vi "Knock Sensor Page Wrapper.vi"(8 "error in (no error)":errorcluster, 11 "Node Ptr":T1 format="%.0x") -> (0 "error out":errorcluster)   [LabVIEW 2015, in "Engine Simulation Toolkit System Explorer.lvlib"]
uses:
  Engine Simulation Toolkit System Explorer.lvlib
  <vilib>/NI Veristand/Custom Device API/Custom Device Item Ref.ctl
  Knock Sensor Page - Multi FPGA.vi
  Knock Sensor Page.vi
  Shared/Properties.vi
  Shared/Engine Simulation Toolkit Shared.lvlib
  <vilib>/NI VeriStand/Custom Device API/Custom Device API.lvlib
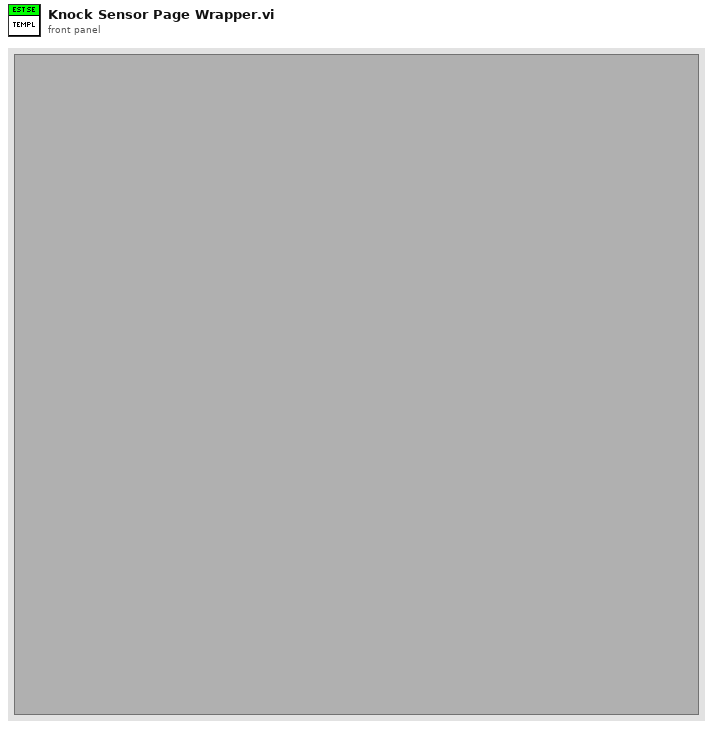
[diagram p1: front panel]
types:
  T1 = typedef "Custom Device API.lvlib/Custom Device Item Ref.ctl" = u64
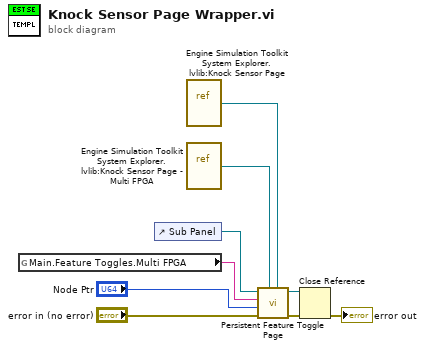
[diagram p0: block diagram]
diagram:
  n1 = global read "Properties.vi" "Main.Feature Toggles.Multi FPGA"() -> (w1:string)
  n2 = control-ref of="Sub Panel"() -> (w7:refnum<vi>)
  n3 = vi-ref "Engine Simulation Toolkit System Explorer.lvlib:Knock Sensor Page.vi"() -> (w6:refnum<vi>)
  n4 = vi-ref "Engine Simulation Toolkit System Explorer.lvlib:Knock Sensor Page - Multi FPGA.vi"() -> (w5:refnum<vi>)
  n5 = call "Persistent Feature Toggle Page.vi"("feature disabled vi"=w6, "feature enabled vi"=w5, "error in (no error)"="error in (no error)", "Node Ptr"="Node Ptr", "property name"=w1, "SubPanel in"=w7) -> ("error out"=w3:errorcluster, "SubPanel out"=w2:refnum<vi>)  [unwired: 4 in]
  n6 = Close Reference(reference=w2, error in (no error)=w3) -> (error out=→"error out":errorcluster)
